vi "maze_v5.vi"   [LabVIEW 2012]
uses:
  <vilib>/NXT/Subs/MotorOutput.ctl
  <vilib>/NXT/Dual Mode Library/Waits/Wait_Num(msec).vi
  <vilib>/NXT/Dual Mode Library/Sound/Tone.vi
types:
  T1 = typedef "MotorOutput.ctl" = u8
  T2 = typedef "LVHSConnector.ctl" = cluster{"Hardware":string, "Flattened String":string}
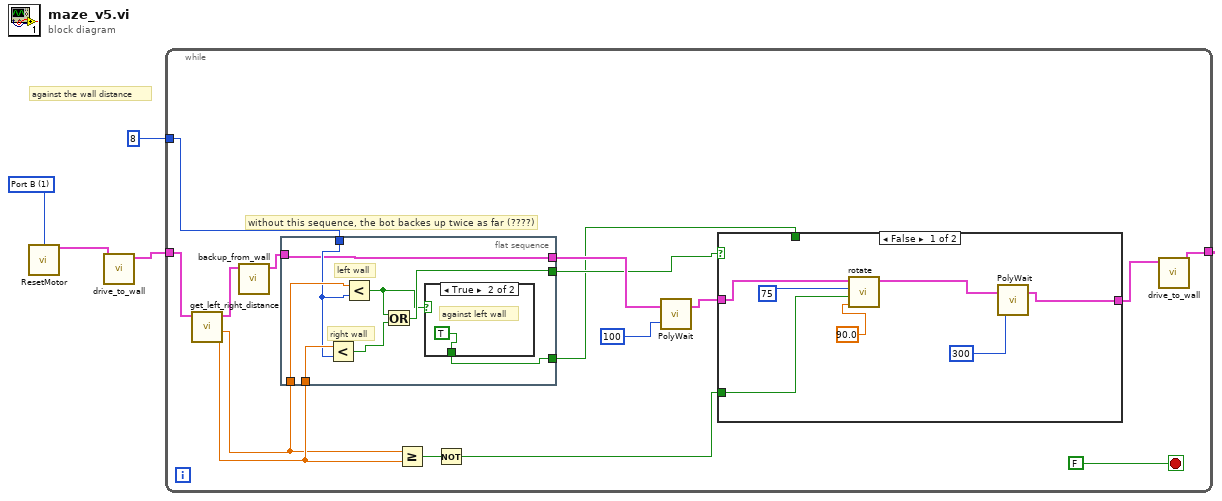
[diagram p0: block diagram]
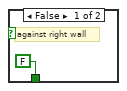
[diagram p2: hidden frame]
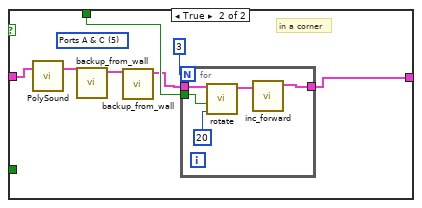
[diagram p3: hidden frame]
diagram:
  w4 = T1 1 items=["Port A"=0, "Port B"=1, "Port C"=2, "Ports A & B"=4, "Ports A & C"=5, "Ports B & C"=6, "All Ports"=3] ("Output Port (All Ports)")
  # "against the wall distance"
  n1 = call <vilib>:"ResetMotor.vi"("Port (All Ports)"=w4) -> ("NXT"=w3:T2)  [unwired: 3 in]
  n2 = call "drive_to_wall.vi"("NXT"=w3) -> ("NXT 2"=w2:T2)  [unwired: 10 in]
  n3 = while {
    tunnel: w2 -> [w20]
    tunnel: u16 8 ("power") -> [w10]
    tunnel: [w15] -> _
    stop <- FALSE stop-if-true
    # "without this sequence, the bot backes up twice as far (????)"
    n4 = call "get_left_right_distance.vi"("NXT"=w20) -> ("right distance"=w11:dbl, "left distance"=w9:dbl, "NXT 2"=w6:T2)  [unwired: 8 in]
    n5 = call "backup_from_wall.vi"("NXT"=w6) -> ("NXT2"=w5:T2)  [unwired: 10 in]
    n6 = flat-sequence {
      tunnel: [w21] -> w14
      tunnel: w11 -> [w28]
      tunnel: w10 -> [w26]
      tunnel: w9 -> [w27]
      tunnel: [w24] -> w8
      tunnel: [w22] -> w7
      tunnel: w5 -> [w21]
      frame #0 {
        # "left wall"
        # "right wall"
        n7 = Less?(x=w28, y=w26) -> (x < y?=w25:bool)
        n8 = Less?(x=w27, y=w26) -> (x < y?=w23:bool)
        n9 = Or(x=w23, y=w25) -> (x .or. y?=w24:bool)
        n10 = case shown="True" w23 {
          tunnel: [FALSE TRUE] -> w22
          frame False {
            # "against right wall"
          }
          frame True {
            # "against left wall"
          }
        }
      }
    }
    n11 = Greater Or Equal?(x=w9, y=w11) -> (x >= y?=w18:bool)
    n12 = Not(x=w18) -> (.not. x?=w17:bool)
    n13 = call-poly <vilib>:"PolyWait.vi"("Time (100 msec)"=u16 100 ("power"), "NXT"=w14) -> ("NXT"=w13:T2)  [unwired: 2 in]
    n14 = case shown="False" w8 {
      tunnel: w7 -> [_ w41]
      tunnel: w13 -> [w32 w38]
      tunnel: [w31 w39] -> w16
      tunnel: w17 -> [w35 _]
      frame False {
        n15 = call "rotate.vi"("degrees to  rotate"=90.0, "right(T)/left(F)"=w35, "power"=u16 75, "NXT 2"=w32) -> ("NXT"=w37:T2)  [unwired: 7 in]
        n16 = call-poly <vilib>:"PolyWait.vi"("Time (100 msec)"=i16 300 ("degrees to  rotate"), "NXT"=w37) -> ("NXT"=w31:T2)  [unwired: 2 in]
      }
      frame True {
        (unwired) T1 5 items=["Port A"=0, "Port B"=1, "Port C"=2, "Ports A & B"=4, "Ports A & C"=5, "Ports B & C"=6, "All Ports"=3] ("Output Port (All Ports)")
        # "in a corner"
        n17 = call-poly <vilib>:"PolySound.vi"("NXT"=w38) -> ("NXT"=w44:T2)  [unwired: 3 in]
        n18 = call "backup_from_wall.vi"("NXT"=w44) -> ("NXT2"=w43:T2)  [unwired: 10 in]
        n19 = call "backup_from_wall.vi"("NXT"=w43) -> ("NXT2"=w40:T2)  [unwired: 10 in]
        n20 = for {
          N: u16 3 ("power") -> [_]
          tunnel: w41 -> [w48]
          tunnel: w40 -> [w47]
          tunnel: [w45] -> w39
          n21 = call "rotate.vi"("degrees to  rotate"=u16 20 ("power"), "right(T)/left(F)"=w48, "NXT 2"=w47) -> ("NXT"=w46:T2)  [unwired: 8 in]
          n22 = call "inc_forward.vi"("NXT"=w46) -> ("NXT2"=w45:T2)  [unwired: 10 in]
        }
      }
    }
    n23 = call "drive_to_wall.vi"("NXT"=w16) -> ("NXT 2"=w15:T2)  [unwired: 10 in]
  }
